vi "PreRegister.vi"(8 "error in (no error)":errorcluster, 11 "VI ref":refnum<vi>) -> (0 "error out":errorcluster, 2 "state":T1(ring), 3 "VI ref":refnum<vi>)   [LabVIEW 2021, in "Autocomplete Textbox.lvlib"]
uses:
  Autocomplete Textbox.lvlib
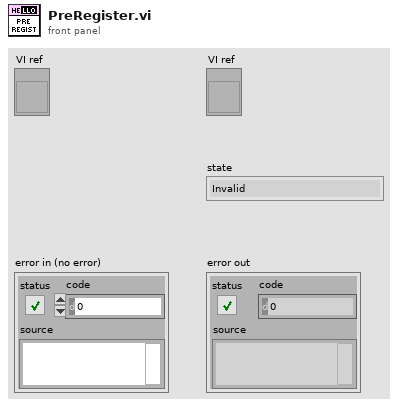
[diagram p1: front panel]
types:
  T1 = enum32{"Invalid", "Standard", "Closed", "Hidden", "Minimized", "Maximized"}
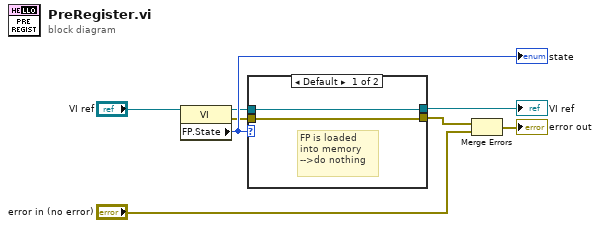
[diagram p0: block diagram]
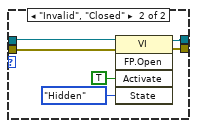
[diagram p2: hidden frame]
diagram:
  n1 = property class="VI"(reference="VI ref") -> (reference out=w3:refnum<vi>, error out=w2:errorcluster, "FP.State"=w5:T1)  [unwired: 1 in]
  "state" <- w5
  n2 = case shown="Default" w5 {
    tunnel: w3 -> [w10 w14]
    tunnel: [w9 w13] -> w8
    tunnel: [w10 w12] -> w6
    tunnel: w2 -> [w9 w11]
    frame Default {
      # "FP is loaded\ninto memory\n-->do nothing"
    }
    frame "Invalid", "Closed" {
      n3 = invoke class="VI" method="FP.Open"(reference=w14, error in=w11, "Activate"=TRUE ("Activate?"), "State"=T1."Hidden") -> (reference out=w12:refnum<vi>, error out=w13:errorcluster)  [unwired: 1 in, 3 out]
    }
  }
  "VI ref" <- w6
  n4 = Merge Errors(w8, "error in (no error)") -> (→"error out":errorcluster)
